vi "ble_rsp_system_get_info.vi"(8 "error in (no error)":errorcluster, 11 "COM Bluegiga in":refnum<visa-resource-name>) -> (0 "error out":errorcluster, 1 "full message package":u8[](array[numeric]), 2 "info":string, 3 "COM Bluegiga out":refnum<visa-resource-name>)   [LabVIEW 2013]
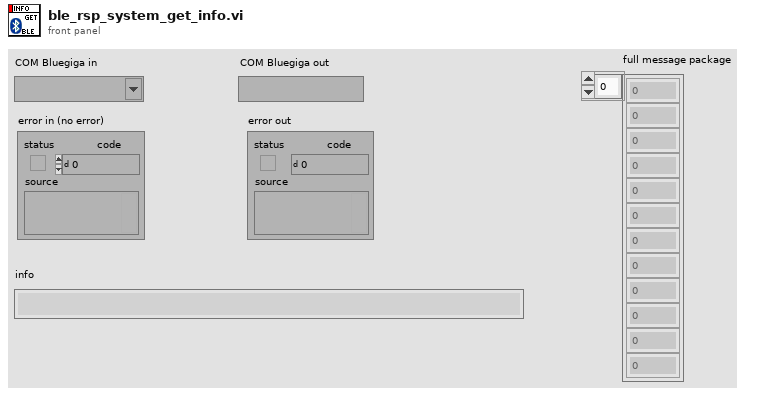
[diagram p1: front panel]
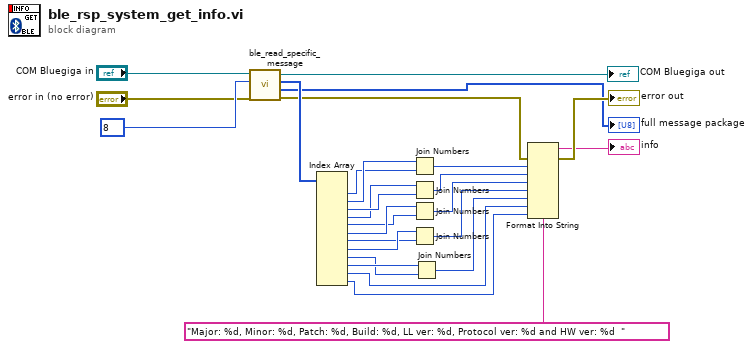
[diagram p0: block diagram]
diagram:
  n1 = call "ble_read_specific_message.vi"("error in (no error)"="error in (no error)", "Message ID (0x00)"=u8 8, "COM Bluegiga in"="COM Bluegiga in") -> ("error out"=w6:errorcluster, "full message package"=→"full message package":u8[], "specific payload"=w25:u8[], "COM Bluegiga out"=→"COM Bluegiga out":refnum<visa-resource-name>)  [unwired: 4 in, 1 out]
  n2 = Index Array(array=w25) -> (element #1=w23:u8, element #2=w24:u8, element #3=w22:u8, element #4=w21:u8, element #5=w19:u8, element #6=w20:u8, element #7=w17:u8, element #8=w18:u8, element #9=w15:u8, element #10=w16:u8, element #11=w8:u8, element #12=w7:u8)  [unwired: 12 in]
  n3 = Join Numbers(hi=w24, lo=w23) -> ((hi.lo)=w13:u16)
  n4 = Join Numbers(hi=w21, lo=w22) -> ((hi.lo)=w12:u16)
  n5 = Join Numbers(hi=w20, lo=w19) -> ((hi.lo)=w11:u16)
  n6 = Join Numbers(hi=w18, lo=w17) -> ((hi.lo)=w10:u16)
  n7 = Join Numbers(hi=w16, lo=w15) -> ((hi.lo)=w9:u16)
  n8 = Format Into String(format string="Major: %d, Minor: %d, Patch: %d, Build: %d, LL ver: %d, Protocol ver: %d and HW ver: %d  ", error in=w6, w13, w12, w11, w10, w9, w8, w7) -> (resulting string=→"info":string, error out=→"error out":errorcluster)  [unwired: 1 in]
